vi "mDrive Send Command.vi"(6 "error in (no error)":errorcluster, 7 "Extra":string, 8 "Command":T1(ring), 9 "VISA resource name":refnum<visa-resource-name>="COM1") -> (0 "error out":errorcluster, 2 "read buffer":string, 3 "VISA resource name out":refnum<visa-resource-name>)   [LabVIEW 2015]
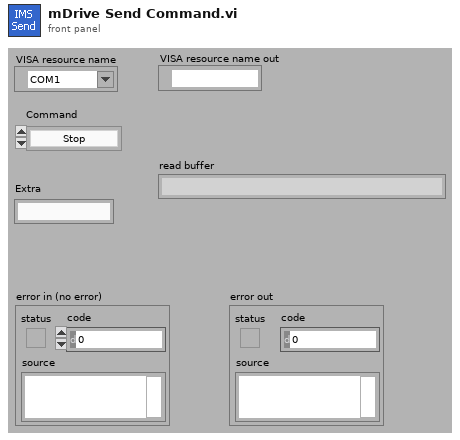
[diagram p1: front panel]
types:
  T1 = enum16{"Stop", "Reset", "Run Current", "Holding Current", "Accel Rate", "Decel Rate", "Move to Relative Position", "Move to Absolute Position", "Echo Mode", "Print Parameter", "Send String", "Microstep Resolution", "Set Current Position", "Max Velocity"}
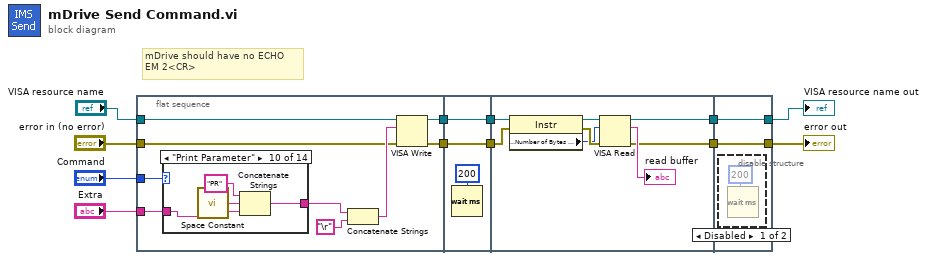
[diagram p0: block diagram]
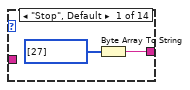
[diagram p2: hidden frame]
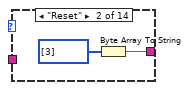
[diagram p3: hidden frame]
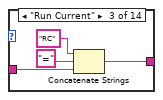
[diagram p4: hidden frame]
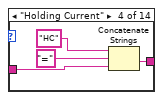
[diagram p5: hidden frame]
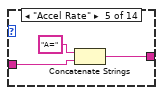
[diagram p6: hidden frame]
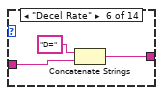
[diagram p7: hidden frame]
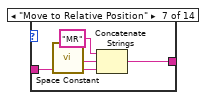
[diagram p8: hidden frame]
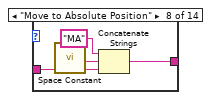
[diagram p9: hidden frame]
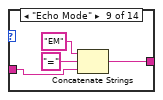
[diagram p10: hidden frame]
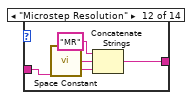
[diagram p12: hidden frame]
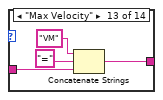
[diagram p13: hidden frame]
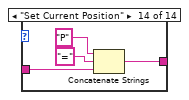
[diagram p14: hidden frame]
diagram:
  # "mDrive should have no ECHO\nEM 2<CR>"
  n1 = flat-sequence {
    tunnel: "Extra" -> [w21]
    tunnel: "Command" -> [w20]
    tunnel: "error in (no error)" -> [w17]
    tunnel: "VISA resource name" -> [w15]
    tunnel: [w14] -> w8
    tunnel: [w13] -> w7
    tunnel: w8 -> [w70]
    tunnel: w7 -> [w69]
    tunnel: [w70] -> w6
    tunnel: [w69] -> w5
    tunnel: w6 -> [w75]
    tunnel: w5 -> [w74]
    tunnel: [w73] -> w2
    tunnel: [w72] -> w1
    tunnel: [w80] -> w4
    tunnel: [w81] -> w3
    tunnel: w2 -> [w81]
    tunnel: w1 -> [w80]
    frame #0 {
      n2 = case shown="\"Print Parameter\"" w20 {
        tunnel: w21 -> [_ _ w27 w31 w34 w38 w41 w45 w48 w52 w56 w57 w62 w66]
        tunnel: [w22 w25 w28 w32 w35 w37 w40 w44 w49 w53 w56 w58 w61 w65] -> w16
        frame "Stop", Default {
          n3 = Byte Array To String(unsigned byte array=u8[] [27]) -> (string=w22:string)
        }
        frame "Reset" {
          n4 = Byte Array To String(unsigned byte array=u8[] [3]) -> (string=w25:string)
        }
        frame "Run Current" {
          n5 = Concatenate Strings("RC", "=", w27) -> (w28:string)
        }
        frame "Holding Current" {
          n6 = Concatenate Strings("HC", "=", w31) -> (w32:string)
        }
        frame "Accel Rate" {
          n7 = Concatenate Strings("A=", w34) -> (w35:string)
        }
        frame "Decel Rate" {
          n8 = Concatenate Strings("D=", w38) -> (w37:string)
        }
        frame "Move to Relative Position" {
          n9 = call <vilib>:"Space Constant.vi"() -> ("String"=w42:string)
          n10 = Concatenate Strings("MR", w42, w41) -> (w40:string)
        }
        frame "Move to Absolute Position" {
          n11 = call <vilib>:"Space Constant.vi"() -> ("String"=w46:string)
          n12 = Concatenate Strings("MA", w46, w45) -> (w44:string)
        }
        frame "Echo Mode" {
          n13 = Concatenate Strings("EM", "=", w48) -> (w49:string)
        }
        frame "Print Parameter" {
          n14 = call <vilib>:"Space Constant.vi"() -> ("String"=w54:string)
          n15 = Concatenate Strings("PR", w54, w52) -> (w53:string)
        }
        frame "Send String" {
        }
        frame "Microstep Resolution" {
          n16 = call <vilib>:"Space Constant.vi"() -> ("String"=w59:string)
          n17 = Concatenate Strings("MR", w59, w57) -> (w58:string)
        }
        frame "Max Velocity" {
          n18 = Concatenate Strings("VM", "=", w62) -> (w61:string)
        }
        frame "Set Current Position" {
          n19 = Concatenate Strings("P", "=", w66) -> (w65:string)
        }
      }
      n20 = Concatenate Strings(w16, "\r") -> (w18:string)
      n21 = VISA Write(VISA resource name=w15, write buffer=w18, error in (no error)=w17) -> (VISA resource name out=w14:refnum<visa-resource-name>, error out=w13:errorcluster)  [unwired: 1 out]
    }
    frame #1 {
      n22 = Wait (ms)(milliseconds to wait=u32 200) -> ()  [unwired: 1 out]
    }
    frame #2 {
      n23 = property class="Instr"(reference=w75, error in=w74) -> (reference out=w78:refnum<visa-resource-name>, error out=w79:errorcluster, "Serial Settings:Number of Bytes at Serial Port"=w77:u32)
      n24 = VISA Read(VISA resource name=w78, byte count=w77, error in (no error)=w79) -> (VISA resource name out=w73:refnum<visa-resource-name>, read buffer=→"read buffer":string, error out=w72:errorcluster)  [unwired: 1 out]
    }
    frame #3 {
      n25 = disable-structure shown="Disabled" {
        frame Disabled {
          n26 = Wait (ms)(milliseconds to wait=u32 200) -> ()  [unwired: 1 out]
        }
        frame Enabled {
        }
      }
    }
  }
  "error out" <- w4
  "VISA resource name out" <- w3
